vi "Aborted funct acq cleanup.vi"(10 "Metadata for all trials/volumes":T1[](array[typedef])=[{"Imaging Protocol"=enum."Functional Acquisition", "Number of Trials"=2, "Frame Size"=512, "# Averaged frames"=1, "Dwell time (us)"=0.1, "Index of Z-plane"=0, "Timelapse?"=FALSE, "Logging process is active"=TRUE, "Speed logging enabled"=FALSE, "tdms file ref"=refnum, "path"=path "E:/UCL/Rig 3 MovCor integration version/Datasets/Dual Plane datasets/150701_01_13_28/Functional imaging TDMS data files/001.tdms", "Trial Number"=1, "Expected # points acquired"=TRUE, "Manually stopped"=FALSE, "Ch0 data"=[], "Ch1 data"=[], "Ref Data"=[], "Last trial"=FALSE, "Ref Dwell time (us)"=0.20000000298023224, "# Ref Averaged frames"=1, "Ref X Length"=0, "Ref Y Length"=0, "Points acquired"={"Ch0 last trial"=34078720, "Ch1 last trial"=34078720, "All trials"=34078720}}, {"Imaging Protocol"=enum."Functional Acquisition", "Number of Trials"=2, "Frame Size"=512, "# Averaged frames"=1, "Dwell time (us)"=0.1, "Index of Z-plane"=0, "Timelapse?"=FALSE, "Logging process is active"=TRUE, "Speed logging enabled"=FALSE, "tdms file ref"=refnum, "path"=path "E:/UCL/Rig 3 MovCor integration version/Datasets/Dual Plane datasets/150701_01_13_28/Functional imaging TDMS data files/002.tdms", "Trial Number"=2, "Expected # points acquired"=TRUE, "Manually stopped"=FALSE, "Ch0 data"=[], "Ch1 data"=[], "Ref Data"=[], "Last trial"=TRUE, "Ref Dwell time (us)"=0.20000000298023224, "# Ref Averaged frames"=1, "Ref X Length"=0, "Ref Y Length"=0, "Points acquired"={"Ch0 last trial"=34078720, "Ch1 last trial"=34078720, "All trials"=68157440}}, {"Imaging Protocol"=enum."Functional Acquisition", "Number of Trials"=2, "Frame Size"=512, "# Averaged frames"=1, "Dwell time (us)"=0.1, "Index of Z-plane"=0, "Timelapse?"=FALSE, "Logging process is active"=TRUE, "Speed logging enabled"=FALSE, "tdms file ref"=refnum, "path"=path "E:/UCL/Rig 3 MovCor integration version/Datasets/Dual Plane datasets/150701_01_13_28/Functional imaging TDMS data files/003.tdms", "Trial Number"=2, "Expected # points acquired"=TRUE, "Manually stopped"=FALSE, "Ch0 data"=[], "Ch1 data"=[], "Ref Data"=[], "Last trial"=TRUE, "Ref Dwell time (us)"=0.20000000298023224, "# Ref Averaged frames"=1, "Ref X Length"=0, "Ref Y Length"=0, "Points acquired"={"Ch0 last trial"=34078720, "Ch1 last trial"=34078720, "All trials"=68157440}}] {"Ref Dwell time (us)" format="%#.6g"; "Frame Size" items=["100X100"=100, "128X128"=128, "200X200"=200, "256X256"=256, "512X512"=512, "1024x1024"=1024, "2048x2048"=2048]; "Dwell time (us)" format="%#.6g"}) -> (0 "error out":errorcluster)   [LabVIEW 2017]
uses:
  Typedefs/Logging queue element.ctl
  Typedefs/Imaging Protocols enum.ctl
  Typedefs/Frame Size.ctl
  Typedefs/Acquired points count.ctl
  Typedefs/Top level VI states.ctl
  Global Variables/General Globals.vi
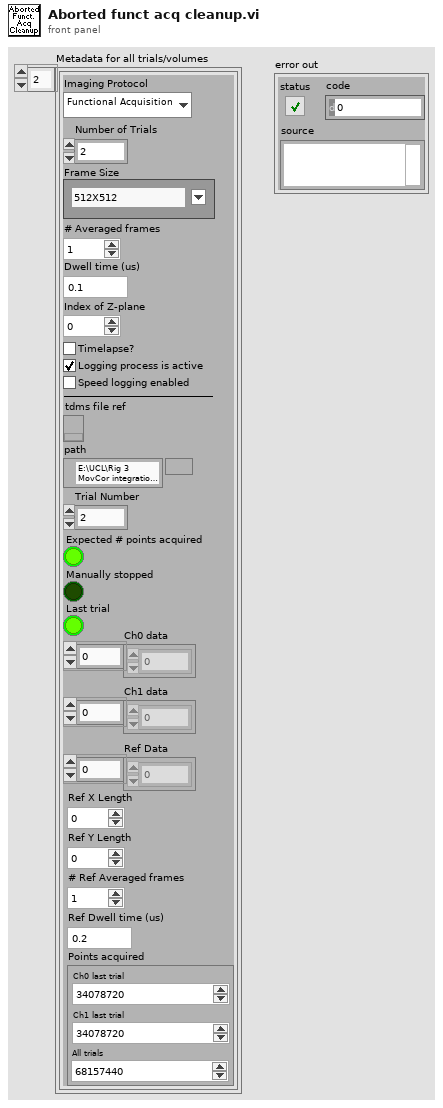
[diagram p1: front panel]
types:
  T1 = typedef "Logging queue element.ctl" = cluster{"Imaging Protocol":T2, "Number of Trials":u16, "Frame Size":T3, "# Averaged frames":u16, "Dwell time (us)":dbl, "Index of Z-plane":i32, "Timelapse?":bool, "Logging process is active":bool, "Speed logging enabled":bool, "tdms file ref":refnum<k34>, "path":path, "Trial Number":i32, "Expected # points acquired":bool, "Manually stopped":bool, "Ch0 data":u32[], "Ch1 data":u32[], "Ref Data":u32[], "Last trial":bool, "Ref Dwell time (us)":dbl, "# Ref Averaged frames":u16, "Ref X Length":u16, "Ref Y Length":u16, "Points acquired":T4}
  T2 = typedef "Imaging Protocols enum.ctl" = enum16{"AOL Z-Stack", "Motor Z Stack", "Functional Acquisition", "Single Plane Acquisition", "Volume Acquisition", "Live Imaging", "Live Plane Imaging", "Live Volume Imaging"}
  T3 = typedef "Frame Size.ctl" = u16
  T4 = typedef "Acquired points count.ctl" = cluster{"Ch0 last trial":u64, "Ch1 last trial":u64, "All trials":u64}
  T5 = typedef "Top level VI states.ctl" = enum16{"None", "Initialise UI", "<STACK PROTOCOL STATES>", "AOL Zstack-START", "AOL Zstack-STOP", "Motor Zstack-START", "Motor Zstack-STOP", "<ACQUISITION PROTOCOL STATES> ", "Functional Acquisition-START", "Functional Acquisition-STOP", "Single Plane Acquisition-START", "Single Plane Acquisition-STOP", "Volume Acquisition-START", "Volume Acquisition-STOP", "<LIVE IMAGING PROTOCOL STATES>", "Live Imaging-START", "Live Imaging-STOP", "Live Plane Imaging-START", "Live Plane Imaging-STOP", "Live Volume Imaging-START", "Live Volume Imaging-STOP", "<MOVEMENT CORRECTION PROTOCOL STATES>", "Background MovCor-START", "Background MovCor-STOP", "EXIT"}
  T6 = enum16{"open", "replace", "create", "open or create", "replace or create", "replace or create with confirmation"}
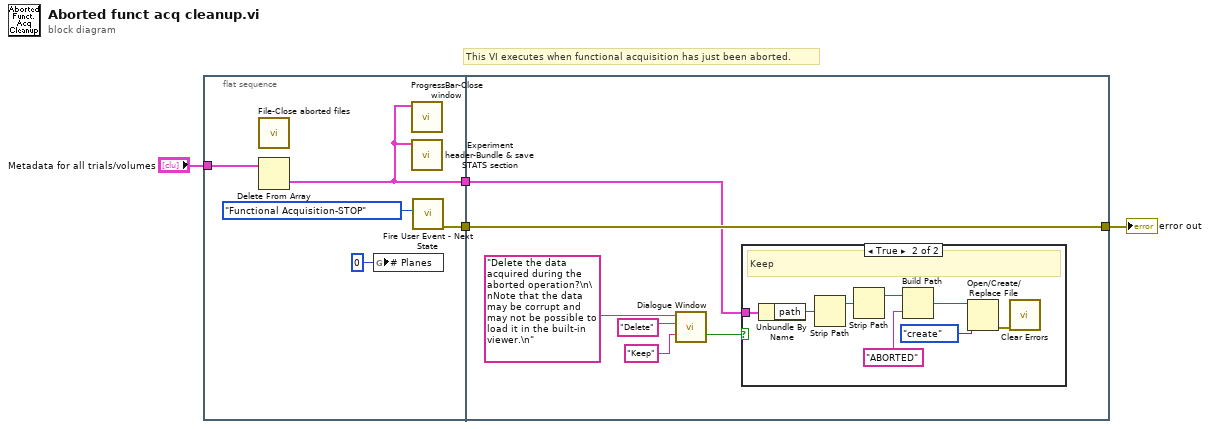
[diagram p0: block diagram]
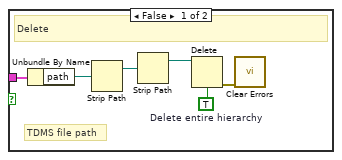
[diagram p2: hidden frame]
diagram:
  # "This VI executes when functional acquisition has just been aborted."
  n1 = flat-sequence {
    tunnel: [w7] -> w4
    tunnel: [w5] -> w3
    tunnel: "Metadata for all trials/volumes" -> [w6]
    tunnel: [w15] -> w2
    tunnel: w4 -> [w15]
    tunnel: w3 -> [w14]
    frame #0 {
      n2 = call "File-Close aborted files.vi"() -> ()  [unwired: 12 in]
      n3 = Delete From Array(array=w6) -> (deleted portion=w5:T1)  [unwired: 2 in, 1 out]
      n4 = global write "General Globals.vi" "# Planes"(0 ("# Planes")) -> ()
      n5 = call "ProgressBar-Close window.vi"("Z-stack queue cluster"=w5) -> ()  [unwired: 10 in, 1 out]
      n6 = call "Experiment header-Bundle & save STATS section.vi"("Logging queue element"=w5) -> ()  [unwired: 10 in, 1 out]
      n7 = call "Fire User Event - Next State.vi"("\"UI Handler loop\" case to execute"=Top_level_VI_states."Functional Acquisition-STOP" ("event data / imaging mode")) -> ("Error Out"=w7:errorcluster)  [unwired: 10 in]
    }
    frame #1 {
      n8 = call "Dialogue Window.vi"("Caption-Left button (Cancel)"="Keep", "Caption-Right button (OK)"="Delete", "Message string"="Delete the data acquired during the aborted operation?\n\nNote that the data may be corrupt and may not be possible to load it in the built-in viewer.\n") -> ("Cancelled (Left button pressed)"=w11:bool)  [unwired: 6 in, 2 out]
      n9 = case shown="True" w11 {
        tunnel: w14 -> [w21 w27]
        frame False {
          w17 = TRUE  # Delete entire hierarchy
          # "TDMS file path"
          # "Delete"
          n10 = Unbundle By Name(w21) -> ("path"=w20:path)
          n11 = Strip Path(path=w20) -> (stripped path=w19:path)  [unwired: 1 out]
          n12 = Strip Path(path=w19) -> (stripped path=w18:path)  [unwired: 1 out]
          n13 = Delete(path (use dialog)=w18, entire hierarchy (F)=w17) -> (error out=w16:errorcluster)  [unwired: 3 in, 2 out]
          n14 = call <vilib>:"Clear Errors.vi"("error in (no error)"=w16) -> ()  [unwired: 5 in, 2 out]
        }
        frame True {
          # "Keep"
          n15 = Unbundle By Name(w27) -> ("path"=w29:path)
          n16 = Strip Path(path=w29) -> (stripped path=w28:path)  [unwired: 1 out]
          n17 = Strip Path(path=w28) -> (stripped path=w26:path)  [unwired: 1 out]
          n18 = Build Path(base path=w26, name or relative path="ABORTED") -> (appended path=w24:path)
          n19 = Open/Create/Replace File(file path (use dialog)=w24, operation (0:open)=T6."create") -> (error out=w22:errorcluster)  [unwired: 4 in, 2 out]
          n20 = call <vilib>:"Clear Errors.vi"("error in (no error)"=w22) -> ()  [unwired: 5 in, 2 out]
        }
      }
    }
  }
  "error out" <- w2
